vi "Write Player Info.vi"(8 "error in (no error)":errorcluster, 10 "Player Info":T1={"Name"="", "Color Box"=0, "Gloat Phrase"="All your base are belong to us!!"}, 11 "Protector in":refnum<class "Protector.lvclass">) -> (0 "error out":errorcluster, 3 "Protector out":refnum<class "Protector.lvclass">)   [LabVIEW 2014, in "Protector.lvclass"]
uses:
  Protector.lvclass
  Player Info.ctl
  Formics/Formics.lvclass
  SquareBattle.lvclass
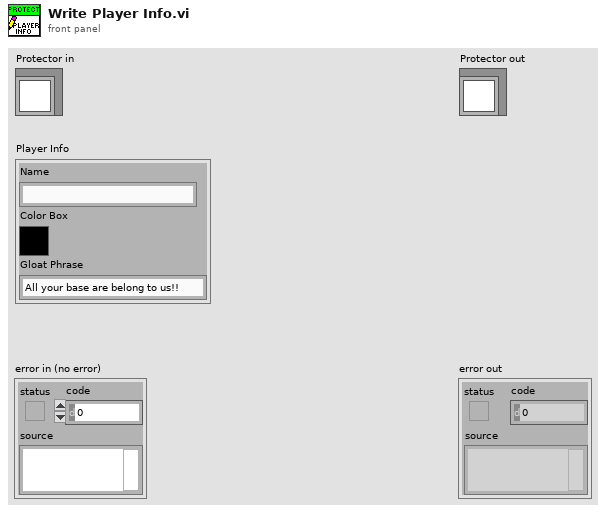
[diagram p1: front panel]
types:
  T1 = typedef "SquareBattle.lvclass/Player Info.ctl" = cluster{"Name":string, "Color Box":u32, "Gloat Phrase":string}
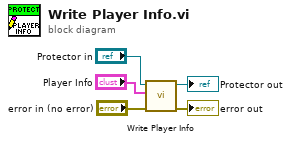
[diagram p0: block diagram]
diagram:
  n1 = call-parent "Write Player Info.vi"("error in (no error)"="error in (no error)", "Player Info"="Player Info", "Mother in"="Protector in") -> ("error out"=→"error out":errorcluster, "Mother out"=→"Protector out":refnum<class "Protector.lvclass">)  [unwired: 7 in]
